vi "Read Config from File.vi"(8 "error in (no error)":errorcluster, 11 "Macro in":refnum<class "Macro.lvclass">) -> (0 "error out":errorcluster, 3 "Macro out":refnum<class "Macro.lvclass">)   [LabVIEW 2020, in "MacroAssert.lvlib" / "Macro.lvclass"]
uses:
  Macro.lvclass
  Macro.lvclass/Macro.ctl
  CTLs/Macro Config V3.ctl
  MacroAssert.lvlib
  <vilib>/Utility/config.llb/NI_LVConfig.lvlib
  <vilib>/Utility/config.llb/Read Key (String).vi
  <vilib>/Utility/config.llb/Read Key (I32).vi
  <vilib>/Utility/config.llb/Read Key (U32).vi
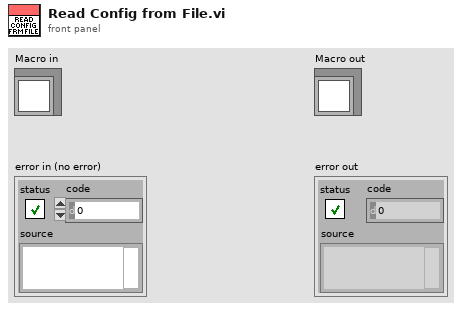
[diagram p1: front panel]
types:
  T1 = typedef "MacroAssert.lvlib/Macro Config V3.ctl" = cluster{"Schema Version":string, "Activation Type":enum32{"Hotkey", "Automatic"}, "N":i32, "Description":string, "Resolutions":cluster{"Width":i16, "Height":i16}[], "Date Created":timestamp, "Date Updated":timestamp}
  T2 = typedef "NI_LVConfig.lvlib/Config Data RefNum.ctl" = refnum<k1>
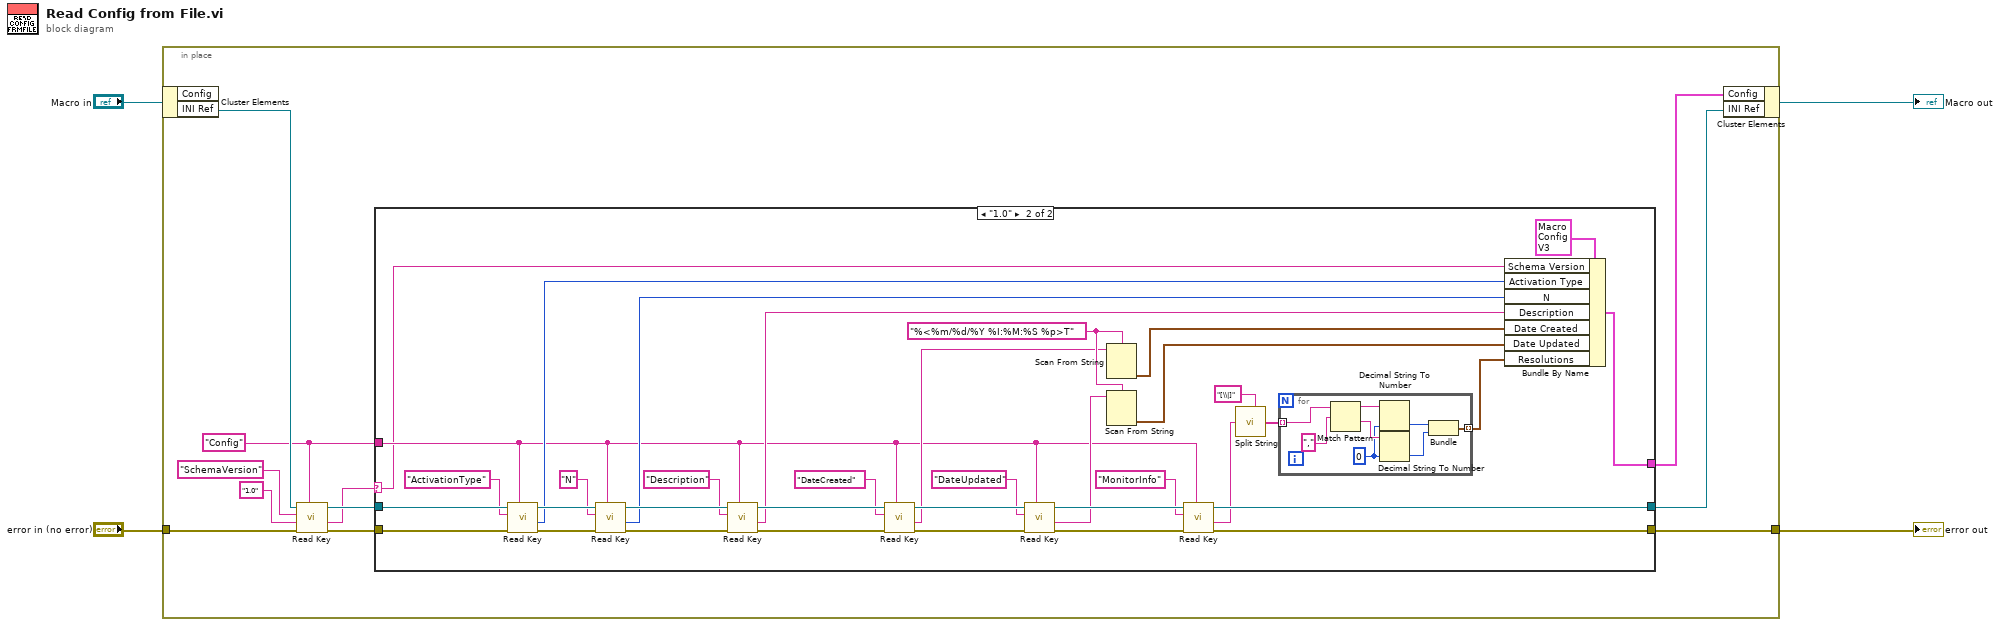
[diagram p0: block diagram]
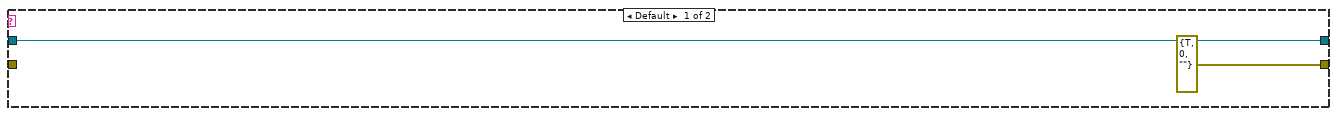
[diagram p2: hidden frame]
diagram:
  n1 = in-place {
    in-place-border: "error in (no error)" -> [w10]
    in-place-border: [w15] -> w3
    w7 = "Config" ("section")
    n2 = in-place-cluster #1("Macro in") -> ("INI Ref"=w8:T2)  [unwired: 1 out]
    n3 = call-poly <vilib>:"Read Key.vi"("section"=w7, "error in (no error)"=w10, "default value"="1.0", "key"="SchemaVersion", "refnum"=w8) -> ("error out"=w9:errorcluster, "value"=w5:string, "refnum out"=w6:T2)  [unwired: 3 in, 1 out]
    n4 = case shown="\"1.0\"" w5 {
      selector: w5 -> [_ w18]
      tunnel: w6 -> [w17 w53]
      tunnel: [w17 w25] -> w13
      tunnel: w9 -> [_ w46]
      tunnel: w7 -> [_ w19]
      tunnel: [errorcluster {"status"=TRUE, "code"=0, "source"=""} ("error out") w24] -> w15
      tunnel: [_ w45] -> w14
      frame Default {
      }
      frame "1.0" {
        w34 = "%<%m/%d/%Y %I:%M:%S %p>T" ("format string")
        n5 = call-poly <vilib>:"Read Key.vi"("section"=w19, "error in (no error)"=w46, "key"="ActivationType", "refnum"=w53) -> ("error out"=w42:errorcluster, "value"=w37:u32, "refnum out"=w52:T2)  [unwired: 4 in, 1 out]
        n6 = call-poly <vilib>:"Read Key.vi"("section"=w19, "error in (no error)"=w42, "key"="N", "refnum"=w52) -> ("error out"=w40:errorcluster, "value"=w36:i32, "refnum out"=w51:T2)  [unwired: 4 in, 1 out]
        n7 = call-poly <vilib>:"Read Key.vi"("section"=w19, "error in (no error)"=w40, "key"="Description", "refnum"=w51) -> ("error out"=w38:errorcluster, "value"=w35:string, "refnum out"=w50:T2)  [unwired: 4 in, 1 out]
        n8 = call-poly <vilib>:"Read Key.vi"("section"=w19, "error in (no error)"=w38, "key"="DateCreated", "refnum"=w50) -> ("error out"=w30:errorcluster, "value"=w28:string, "refnum out"=w49:T2)  [unwired: 4 in, 1 out]
        n9 = call-poly <vilib>:"Read Key.vi"("section"=w19, "error in (no error)"=w30, "key"="DateUpdated", "refnum"=w49) -> ("error out"=w26:errorcluster, "value"=w27:string, "refnum out"=w48:T2)  [unwired: 4 in, 1 out]
        n10 = Scan From String(format string=w34, input string=w28) -> (output 1=w33:timestamp)  [unwired: 3 in, 3 out]
        n11 = Scan From String(format string=w34, input string=w27) -> (output 1=w32:timestamp)  [unwired: 3 in, 3 out]
        n12 = call-poly <vilib>:"Read Key.vi"("section"=w19, "error in (no error)"=w26, "key"="MonitorInfo", "refnum"=w48) -> ("error out"=w24:errorcluster, "value"=w21:string, "refnum out"=w25:T2)  [unwired: 4 in, 1 out]
        n13 = call <vilib>:"Split String.vi"("Split Pattern"="[\\|]", "Input String"=w21) -> ("Split String"=w23:string[])  [unwired: 5 in]
        n14 = for {
          tunnel: w23 -> [w61] mode=indexing
          tunnel: [w55] -> w20 mode=indexing
          w54 = i16 0 ("default (0 I32)")
          n15 = Match Pattern(string=w61, regular expression=",") -> (before substring=w59:string, after substring=w58:string)  [unwired: 1 in, 2 out]
          n16 = Decimal String To Number(string=w59, default (0L)=w54) -> (number=w57:i16)  [unwired: 1 in, 1 out]
          n17 = Decimal String To Number(string=w58, default (0L)=w54) -> (number=w56:i16)  [unwired: 1 in, 1 out]
          n18 = Bundle(w57, w56) -> (w55:cluster{i16, i16})  [unwired: 1 in]
        }
        n19 = Bundle By Name(cluster=T1 {"Schema Version"="", "Activation Type"=enum."Hotkey", "N"=0, "Description"="", "Resolutions"=[], "Date Created"=timestamp(0 s since 1904-01-01), "Date Updated"=timestamp(0 s since 1904-01-01)} ("Macro Config"), "Schema Version"=w18, "Activation Type"=w37, "N"=w36, "Description"=w35, "Date Created"=w33, "Date Updated"=w32, "Resolutions"=w20) -> (w45:T1)
      }
    }
    n20 = in-place-cluster #1("Config"=w14, "INI Ref"=w13) -> (→"Macro out":refnum<class "Macro.lvclass">)
  }
  "error out" <- w3
